vi "Add Connection.vi"(8 "error in (no error)":errorcluster, 9 "remote address":string, 10 "connection ID":refnum<k5>, 11 "ServerListener in":refnum<class "ServerListener.lvclass">) -> (0 "error out":errorcluster, 3 "ServerListener out":refnum<class "ServerListener.lvclass">)   [LabVIEW 2026, in "ServerListener.lvlib" / "ServerListener.lvclass"]
uses:
  ServerListener.lvclass
  C:/Program Files/National Instruments/LabVIEW 2026/vi.lib/ActorFramework/Actor/Actor.lvclass
  <vilib>/ActorFramework/Actor/Actor.lvclass/Actor.ctl
  Client Proxy LNA/Client Proxy LNA.lvclass/Client Proxy LNA.ctl
  Controller/Messages/Launch New Client Proxy Msg/Launch New Client Proxy Msg.lvclass/Launch New Client Proxy Msg.ctl
  <vilib>/ActorFramework/Message Enqueuer/Message Enqueuer.lvclass/Message Enqueuer.ctl
  <vilib>/ActorFramework/Message Enqueuer/Enqueue.vi
  Controller/Messages/Launch New Client Proxy Msg/Launch New Client Proxy Msg.lvclass
  C:/Program Files/National Instruments/LabVIEW 2026/vi.lib/ActorFramework/Message/Message.lvclass
  <vilib>/ActorFramework/Message Priority Queue/Priority Enqueue.vi
  <vilib>/ActorFramework/Actor/Actor.lvclass
  MAL-Framework/user.lib/Common Components/Controller/Messages/Log Status/Log Status.lvclass
  Client Proxy LNA/Client Proxy LNA.lvclass
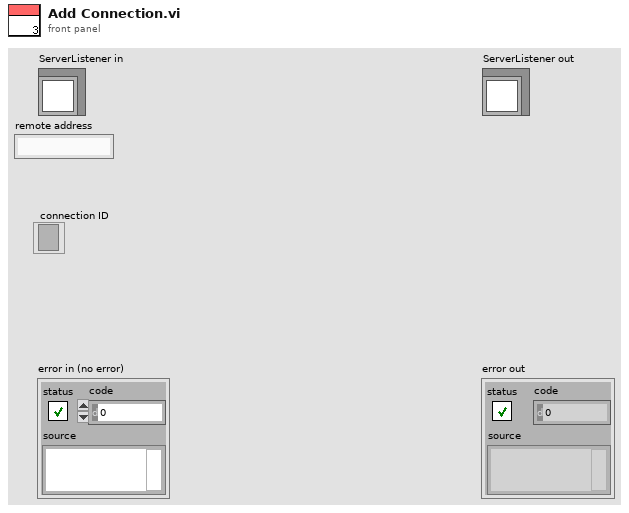
[diagram p1: front panel]
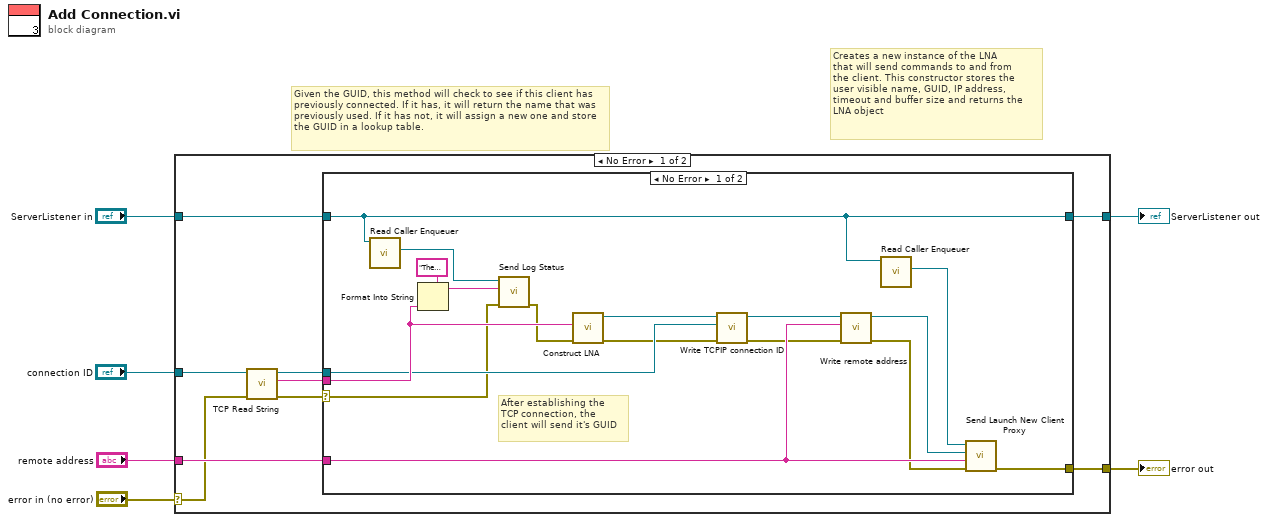
[diagram p0: block diagram]
diagram:
  # "Creates a new instance of the LNA\nthat will send commands to and from\nthe client. This constructor stores the\nuser visible name, GUID, IP address, \ntimeout and buffer size and returns the \nLNA object"
  # "Given the GUID, this method will check to see if this client has previously connected. If it has, it will return the name that was previously used. If it has not, it will assign a new one and store the GUID in a lookup table."
  n1 = case shown="No Error" "error in (no error)" {
    selector: "error in (no error)" -> [w12 w36]
    tunnel: [w10 w36] -> w5
    tunnel: [w7 w35] -> w3
    tunnel: "ServerListener in" -> [w9 w35]
    tunnel: "connection ID" -> [w15 _]
    tunnel: "remote address" -> [w14 _]
    frame No Error {
      n2 = call "TCP Read String.vi"("error in (no error)"=w12, "connection ID"=w15) -> ("error out"=w8:errorcluster, "data out"=w13:string, "connection ID out"=w11:refnum<k5>)  [unwired: 7 in]
      n3 = case shown="No Error" w8 {
        selector: w8 -> [w23 w34]
        tunnel: w14 -> [w20 _]
        tunnel: w13 -> [w29 _]
        tunnel: w11 -> [w27 _]
        tunnel: [w26 w34] -> w10
        tunnel: w9 -> [w16 w33]
        tunnel: [w16 w33] -> w7
        frame No Error {
          # "After establishing the\nTCP connection, the \nclient will send it's GUID"
          n4 = call <vilib>:"Read Caller Enqueuer.vi"("Actor"=w16) -> ("Caller Enqueuer"=w25:refnum<class "Message Enqueuer.lvclass">)  [unwired: 10 in]
          n5 = Format Into String(format string="The listner has received a request for a new connection from %s" ("string"), w29) -> (resulting string=w30:string)  [unwired: 2 in, 1 out]
          n6 = call "Send Log Status.vi"("error in (no error)"=w23, "String"=w30, "Message Enqueuer in"=w25) -> ("error out"=w24:errorcluster)  [unwired: 7 in, 1 out]
          n7 = call "Construct LNA.vi"("error in (no error)"=w24, "Client GUID"=w29) -> ("error out"=w19:errorcluster, "Client Proxy LNA out"=w28:refnum<class "Client Proxy LNA.lvclass">)  [unwired: 8 in]
          n8 = call "Write TCPIP connection ID.vi"("error in (no error)"=w19, "TCPIP connection ID"=w27, "Client Proxy LNA in"=w28) -> ("error out"=w18:errorcluster, "Client Proxy LNA out"=w22:refnum<class "Client Proxy LNA.lvclass">)  [unwired: 7 in]
          n9 = call "Write remote address.vi"("error in (no error)"=w18, "remote address"=w20, "Client Proxy LNA in"=w22) -> ("error out"=w17:errorcluster, "Client Proxy LNA out"=w21:refnum<class "Client Proxy LNA.lvclass">)  [unwired: 7 in]
          n10 = call <vilib>:"Read Caller Enqueuer.vi"("Actor"=w16) -> ("Caller Enqueuer"=w32:refnum<class "Message Enqueuer.lvclass">)  [unwired: 10 in]
          n11 = call "Send Launch New Client Proxy.vi"("error in (no error)"=w17, "remote address"=w20, "Client Proxy LNA"=w21, "Message Enqueuer"=w32) -> ("error out"=w26:errorcluster)  [unwired: 6 in, 1 out]
        }
        frame Error {
        }
      }
    }
    frame Error {
    }
  }
  "error out" <- w5
  "ServerListener out" <- w3
